vi "FR Calculate Fit.vi"(8 "error in (no error)":errorcluster, 10 "FR measurement":T1={"Measurement frequencies (Hz)"=[1000.0, 10000.0, 1000.0], "Sampling frequency (Hz)"=500000.0, "Signal amplitude (V)"=4.5, "AC-DC settle time (s)"=20.0, "Record length (multiples of period)"=[1000.0, 10000.0, 1000.0], "Measurement template file"=path "", "Row of START keyword"=0, "Row of STOP keyword"=0, "Calculate RMS from samples"=FALSE, "AC-DC warm up time (s)"=300.0, "Measurement template line"=[], "DC meter readings No."=10, "Algorithm"="TWM-WFFT", "Simultaneous measurement"=FALSE, "Recalculate-skip already calculated"=FALSE} {"Record length (multiples of period)" format="%#_3p"; "Sampling frequency (Hz)" format="%#_3p"; "Measurement frequencies (Hz)" format="%#_3p"}, 11 "Common properties":T2={"Measurement status ref"=refnum, "TWM Status ref"=refnum, "Abort ref"=refnum, "Skip waiting ref"=refnum, "GNU Octave path"=path "C:/Program Files/GNU Octave/Octave-6.2.0/mingw64/bin", "TWM+QWTB path"=path "C:/Users/labina/Desktop/TWM-1.8.7.0-full/octprog", "lvlib path"=path "D:/martin/WAC/WACsw - github/control_software/Filter function meter/external libraries/GOLPI 0.7.3.1 source distribution LV 20.0 32 bit/lv_proc.dll", "TWM pipe"="\\\\.\\pipe\\TWM:server", "PJVS status ref"=refnum, "WAC path"=path ""}) -> (0 "error out":errorcluster)   [LabVIEW 2020]
doc: "Runs calculation of FR measurement using read_M_FR_from_spreadsheet.m and P_FR.m scripts."
uses:
  Utilities/Type definitions/Common properties.ctl
  FR Measurement/Type definitions/FR measuement.ctl
  Utilities/Calculation related/Globals for GOLPI.vi
  external libraries/GOLPI 0.7.3.1 source distribution LV 20.0 32 bit/GOLPI library.lvlib
panel:
  out "command\n(for debug)":string="addpath('info'); addpath('qwtb'); qwtb_exec_algorithm('%s', 0, 1); disp('FINISHEDCR')"
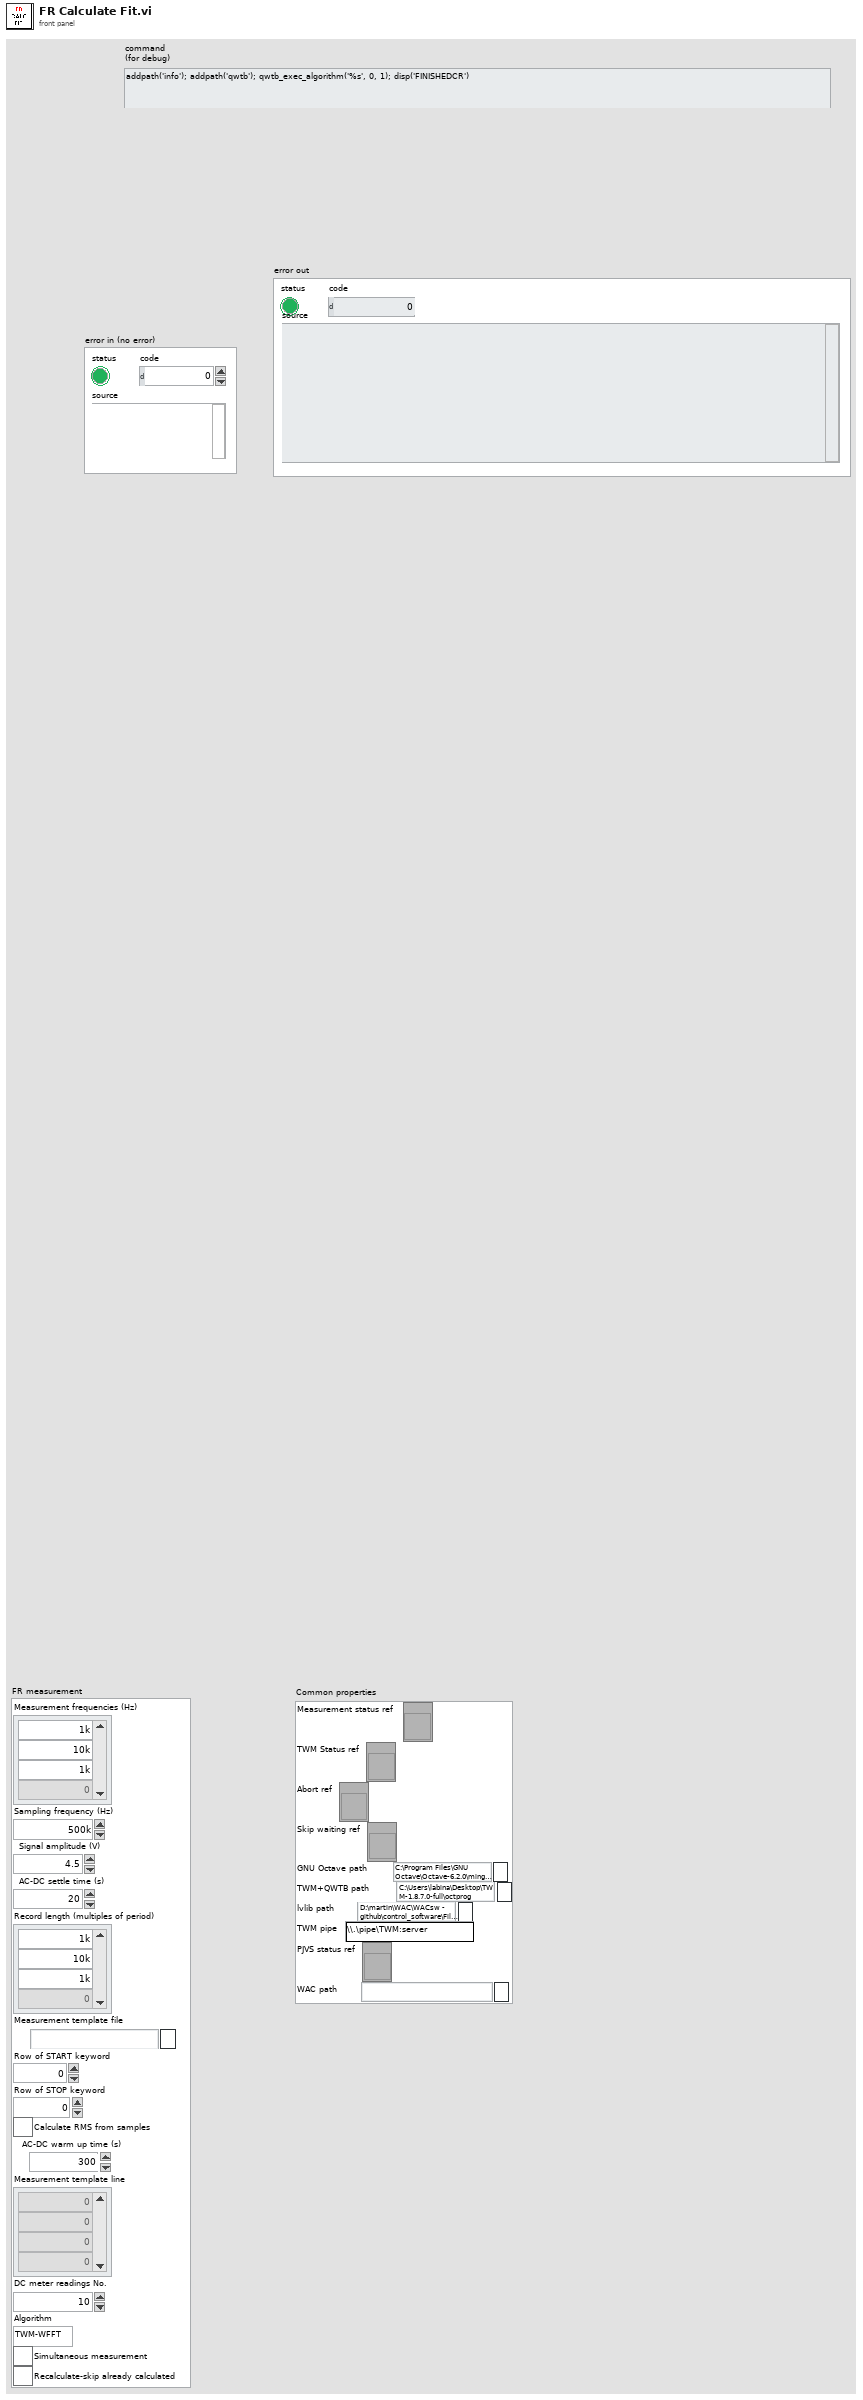
[diagram p1: front panel]
types:
  T1 = typedef "FR measuement.ctl" = cluster{"Measurement frequencies (Hz)":dbl[], "Sampling frequency (Hz)":dbl, "Signal amplitude (V)":dbl, "AC-DC settle time (s)":dbl, "Record length (multiples of period)":dbl[], "Measurement template file":path, "Row of START keyword":i32, "Row of STOP keyword":i32, "Calculate RMS from samples":bool, "AC-DC warm up time (s)":dbl, "Measurement template line":i32[], "DC meter readings No.":i32, "Algorithm":string, "Simultaneous measurement":bool, "Recalculate-skip already calculated":bool}
  T2 = typedef "Common properties.ctl" = cluster{"Measurement status ref":refnum<vi>, "TWM Status ref":refnum<vi>, "Abort ref":refnum<vi>, "Skip waiting ref":refnum<vi>, "GNU Octave path":path, "TWM+QWTB path":path, "lvlib path":path, "TWM pipe":string, "PJVS status ref":refnum<vi>, "WAC path":path}
  T3 = typedef "GOLPI library.lvlib/GOLPI reference Type Def.ctl" = cluster{"pipe handle":T4, "fast read timeout [ms]":u32, "fast read settle time [ms]":u32, "fast read to multiple [ms]":u32, "max elements per input line":u32, "slow read timeout [ms]":u32, "stdin double format specifier":string, "max elements per stdout output column":u32, "console mode bitstream":bool, "bitstream first read timeout [ms]":u32, "bitstream read timeout [ms]":u32, "struct transfer possible":bool, "matlab mode":bool}
  T4 = typedef "LV Process library.lvlib/Pipe Handle.ctl" = cluster{"lv_proc.dll file path":path, "process instance handle":u32[], "debug mode":bool, "debug data":cluster{"time":timestamp, "stdin":bool, "data":string}[]}
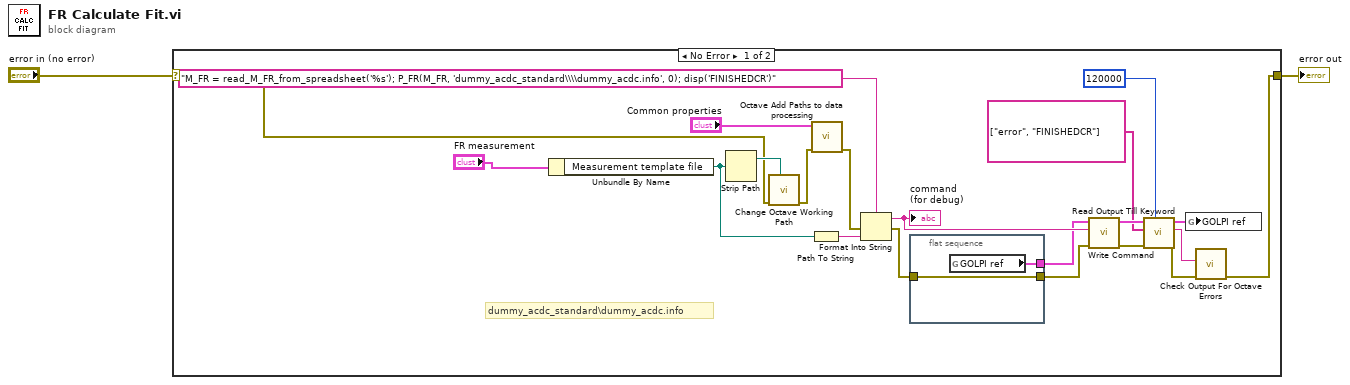
[diagram p0: block diagram]
diagram:
  n1 = case shown="No Error" "error in (no error)" {
    selector: "error in (no error)" -> [w15 w26]
    tunnel: [w3 w26] -> w2
    frame No Error {
      # "dummy_acdc_standard\\dummy_acdc.info"
      n2 = Unbundle By Name("FR measurement") -> ("Measurement template file"=w14:path)
      n3 = Strip Path(path=w14) -> (stripped path=w16:path)  [unwired: 1 out]
      n4 = call "Change Octave Working Path.vi"("Measurement path in"=w16, "error in (no error)"=w15) -> ("error out"=w9:errorcluster)  [unwired: 9 in]
      n5 = Path To String(path=w14) -> (string=w22:string)
      n6 = call "Octave Add Paths to data processing.vi"("error in (no error)"=w9, "Common properties"="Common properties") -> ("error out"=w8:errorcluster)  [unwired: 9 in]
      n7 = Format Into String(format string="M_FR = read_M_FR_from_spreadsheet('%s'); P_FR(M_FR, 'dummy_acdc_standard\\\\dummy_acdc.info', 0); disp('FINISHEDCR')", error in=w8, w22) -> (resulting string=w17:string, error out=w13:errorcluster)  [unwired: 1 in]
      "command\n(for debug)" <- w17
      n8 = flat-sequence {
        tunnel: [w25] -> w12
        tunnel: w13 -> [w25]
        tunnel: [w24] -> w11
        frame #0 {
          n9 = global read "Globals for GOLPI.vi" "GOLPI ref"() -> (w24:T3)
        }
      }
      n10 = call "Write Command.vi"("error in"=w12, "command"=w17, "GOLPI ref. in"=w11) -> ("error out"=w21:errorcluster, "GOLPI ref. out"=w20:T3)  [unwired: 7 in]
      n11 = call "Read Output Till Keyword.vi"("timeout [ms]"=u32 120000, "error in"=w21, "keywords"=string[] ["error", "FINISHEDCR"], "GOLPI ref. in"=w20) -> ("error out"=w4:errorcluster, "read buffer"=w5:string, "GOLPI ref. out"=w10:T3)  [unwired: 4 in, 1 out]
      n12 = global write "Globals for GOLPI.vi" "GOLPI ref"(w10) -> ()
      n13 = call "Check Output For Octave Errors.vi"("error in"=w4, "read buffer"=w5) -> ("error out"=w3:errorcluster)  [unwired: 9 in]
    }
    frame Error {
    }
  }
  "error out" <- w2
